vi "Collector motor.vi"(11 "Collector motor":bool) -> ()   [LabVIEW 2017]
uses:
  Robot Global Data.vi
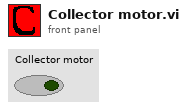
[diagram p1: front panel]
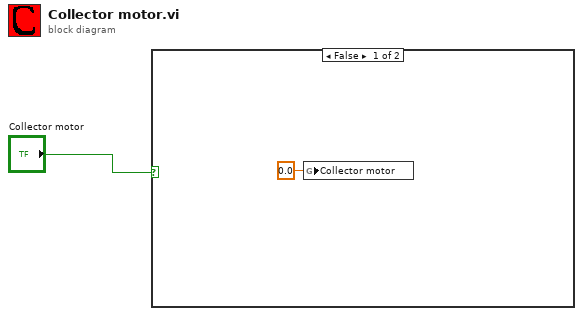
[diagram p0: block diagram]
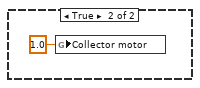
[diagram p2: hidden frame]
diagram:
  n1 = case shown="False" "Collector motor" {
    frame False {
      n2 = global write "Robot Global Data.vi" "Collector motor"(0.0 ("Collector motor")) -> ()
    }
    frame True {
      n3 = global write "Robot Global Data.vi" "Collector motor"(1.0 ("Collector motor")) -> ()
    }
  }
